vi "Wait until Done.vi"(8 "error in (no error)":errorcluster, 10 "timeout [s]":dbl=-1.0, 11 "Analog output in":refnum<class "Analog output.lvclass">) -> (0 "error out":errorcluster, 3 "Analog output out":refnum<class "Analog output.lvclass">)   [LabVIEW 2009, in "MicroDAQ.lvlib" / "Analog output.lvclass"]
uses:
  <instrlib>/MicroDAQ/Channel/Analog Output/Analog output.lvclass
  <instrlib>/MicroDAQ/Channel/Channel.lvclass
  <instrlib>/MicroDAQ/Mlink library wraper/mlink.lvlib
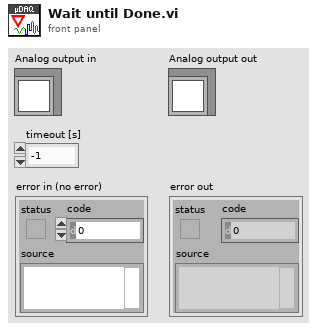
[diagram p1: front panel]
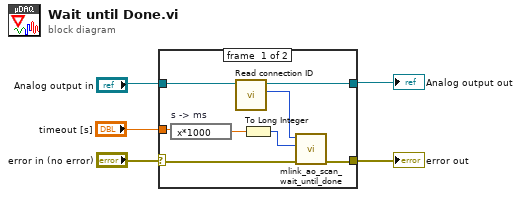
[diagram p0: block diagram]
diagram:
  n1 = case shown="No Error" "error in (no error)" {
    selector: "error in (no error)" -> [w10 w14]
    tunnel: [w11 w14] -> w4
    tunnel: "Analog output in" -> [w13 w15]
    tunnel: [w12 w15] -> w5
    tunnel: "timeout [s]" -> [w7 _]
    frame #0 {
      n2 = expression code="x*1000" "s -> ms"(w7) -> (w8:dbl)
      n3 = call <instrlib>:"Read connection ID.vi"("Task in"=w13) -> ("connection ID"=w9:i32, "Task out"=w12:refnum<class "Analog output.lvclass">)  [unwired: 9 in]
      n4 = To Long Integer(number=w8) -> (32bit integer=w6:i32)
      n5 = call <instrlib>:"mlink_ao_scan_wait_until_done.vi"("error in (no error)"=w10, "timeout"=w6, "connection ID"=w9) -> ("error out"=w11:errorcluster)  [unwired: 7 in, 1 out]
    }
    frame #1 {
    }
  }
  "error out" <- w4
  "Analog output out" <- w5
